vi "系统状态.vi"(1 "状态内容":string) -> (0 "连接的字符串":string)   [LabVIEW 2019]
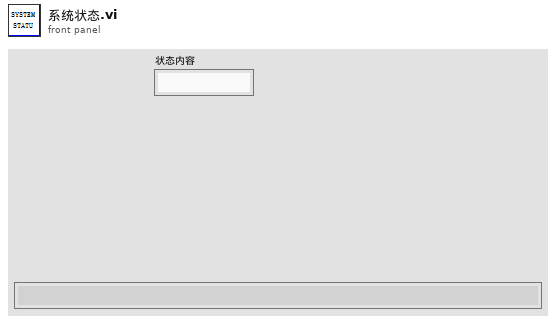
[diagram p1: front panel]
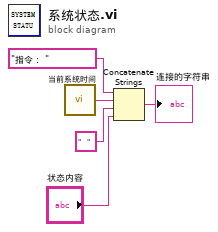
[diagram p0: block diagram]
diagram:
  n1 = call "当前系统时间.vi"() -> ("日期/时间字符串"=w5:string)
  n2 = Concatenate Strings("指令： " ("字符串"), w5, "   " ("字符串"), "状态内容") -> (→"连接的字符串":string)
